vi "Abort If Not Refnum.vi"(8 "error in (no error)":errorcluster, 11 "VI in":refnum<vi>) -> (0 "error out":errorcluster)   [LabVIEW 2013]
doc: "This VI aborts a VI if it is a valid refnum and ignores the error that arises if it is not running."
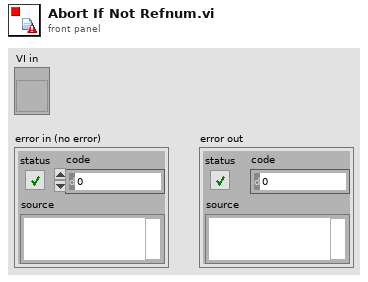
[diagram p1: front panel]
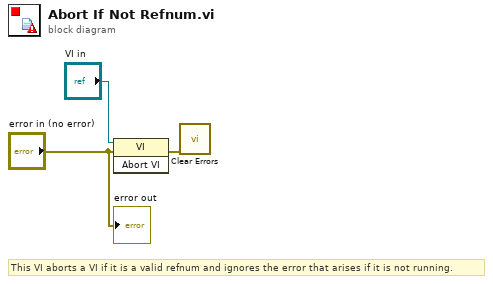
[diagram p0: block diagram]
diagram:
  # "This VI aborts a VI if it is a valid refnum and ignores the error that arises if it is not running."
  n1 = invoke class="VI" method="Abort VI"(reference="VI in", error in="error in (no error)") -> (error out=w2:errorcluster)  [unwired: 1 in, 2 out]
  n2 = call <vilib>:"Clear Errors.vi"("error in (no error)"=w2) -> ()  [unwired: 6 in, 1 out]
  "error out" <- "error in (no error)"
